vi "ShutDownSD.vi"(2 "error in (no error)":errorcluster) -> (0 "error out":errorcluster, 1 "DLL error code":u32)   [LabVIEW 2015]
doc: "This function will close the AndorMCD[tm] system down.\n\n<B>Error code:</B>\nDRV_SUCCESS - System shut down.\n\n<B>NOTES:</B>\n<B>The temperature of the detector should be above zero degrees before shutting down the system.</B>"
uses:
  DLL/atmcd32d.dll
panel:
  out "DLL error code 2":u32
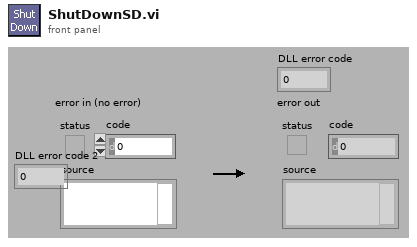
[diagram p1: front panel]
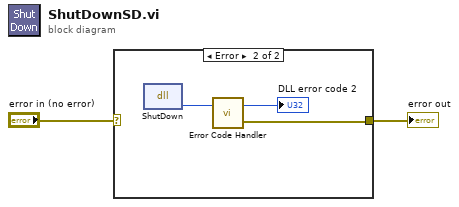
[diagram p0: block diagram]
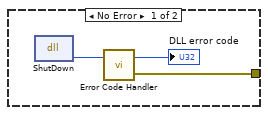
[diagram p2: hidden frame]
diagram:
  n1 = case shown="Error" "error in (no error)" {
    tunnel: [w4 w6] -> w1
    frame No Error {
      n2 = dll-call lib="G:/SD/TRANCON-2015/DLL/Atmcd32d.dll" fn="ShutDown"() -> (w5:u32)  [unwired: 3 in, 2 out]
      n3 = call "Error Code Handler.vi"("DLL error code"=w5) -> ("error out"=w4:errorcluster, "dup DLL error code"=→"DLL error code":u32)  [unwired: 1 out]
    }
    frame Error {
      n4 = dll-call lib="G:/SD/TRANCON-2015/DLL/Atmcd32d.dll" fn="ShutDown"() -> (w8:u32)  [unwired: 3 in, 2 out]
      n5 = call "Error Code Handler.vi"("DLL error code"=w8) -> ("error out"=w6:errorcluster, "dup DLL error code"=→"DLL error code 2":u32)  [unwired: 1 out]
    }
  }
  "error out" <- w1
